vi "Re-Range.vi"(8 "error in (no error)":errorcluster, 10 "Config in":T1, 11 "DMM Driver in":refnum<class "DMM Driver.lvclass">) -> (0 "error out":errorcluster, 1 "Success?":bool, 2 "Config out":T1, 3 "DMM Driver out":refnum<class "DMM Driver.lvclass">)   [LabVIEW 2020, in "DMM.lvlib" / "DMM Driver.lvclass"]
doc: "Re-range the DMM using autorange and single measure. The autoranged measurement is discarded."
uses:
  DMM Driver.lvclass
  Controls/Ctl_DigitResolution.ctl
  DMM.lvlib
  Controls/Ctl_Function.ctl
  Controls/Community/Ctl_Config.ctl
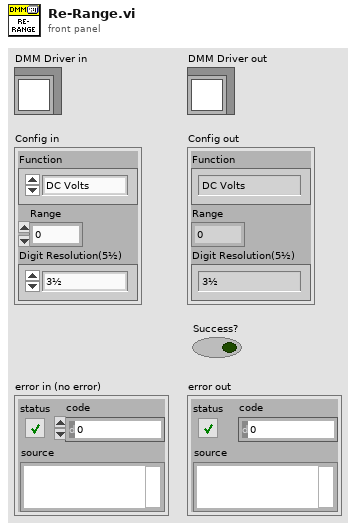
[diagram p1: front panel]
types:
  T1 = typedef "DMM.lvlib/Ctl_Config.ctl" = cluster{"Function":T2, "Range":dbl, "Digit Resolution(5½)":T3}
  T2 = typedef "DMM.lvlib/Ctl_Function.ctl" = enum8{"DC Volts", "AC Volts", "DC Current", "AC Current", "2-wire Resistance", "4-wire Resistance", "Diode", "Frequency", "Period", "AC Volts DC Coupled", "Capacitance", "Inductance", "Temperature"}
  T3 = typedef "DMM.lvlib/Ctl_DigitResolution.ctl" = enum8{"3½", "4½", "5½", "6½", "7½"}
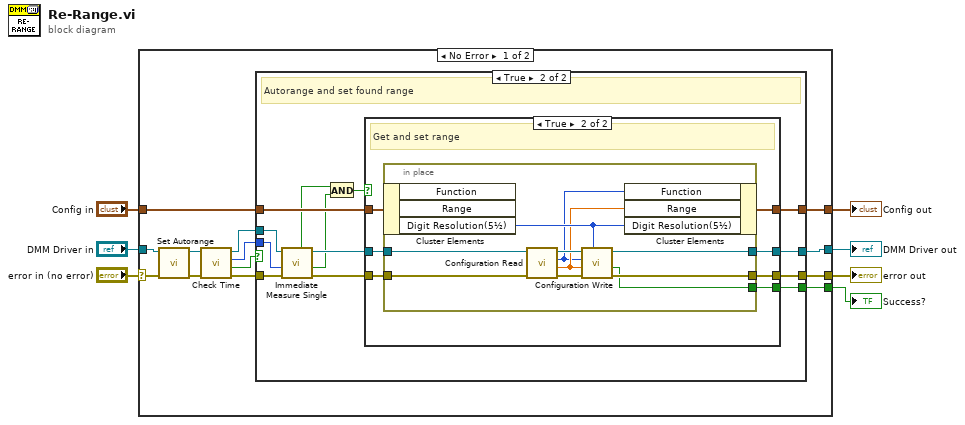
[diagram p0: block diagram]
diagram:
  n1 = case shown="No Error" "error in (no error)" {
    selector: "error in (no error)" -> [w18 w58]
    tunnel: [w20 w59] -> w7
    tunnel: "Config in" -> [w19 w59]
    tunnel: "DMM Driver in" -> [w17 w57]
    tunnel: [w16 _] -> w3
    tunnel: [w15 w57] -> w2
    tunnel: [w14 w58] -> w1
    frame No Error {
      n2 = call-dynamic "Set Autorange.vi"("error in (no error)"=w18, "DMM Driver in"=w17) -> ("error out"=w11:errorcluster, "DMM Driver out"=w8:refnum<class "DMM Driver.lvclass">)  [unwired: 8 in]
      n3 = call "Check Time.vi"("error in (no error)"=w11, "DMM Driver in"=w8) -> ("error out"=w10:errorcluster, "Time OK?"=w12:bool, "Remaining Time"=w13:i32, "DMM Driver out"=w9:refnum<class "DMM Driver.lvclass">)  [unwired: 6 in]
      n4 = case shown="True" w12 {
        tunnel: w9 -> [w22 w36]
        tunnel: w10 -> [w23 w35]
        tunnel: w13 -> [_ w34]
        tunnel: [w23 w31] -> w14
        tunnel: [w22 w30] -> w15
        tunnel: [_ w29] -> w16
        tunnel: w19 -> [w21 w28]
        tunnel: [w21 w27] -> w20
        frame False {
          # "Out of Time"
        }
        frame True {
          # "Autorange and set found range"
          n5 = call-dynamic "Immediate Measure Single.vi"("error in (no error)"=w35, "Max Time (-1ms)"=w34, "DMM Driver in"=w36) -> ("error out"=w32:errorcluster, "Valid measurement?"=w25:bool, "DMM Driver out"=w33:refnum<class "DMM Driver.lvclass">, "Finished?"=w26:bool)  [unwired: 4 in, 1 out]
          n6 = And(x=w26, y=w25) -> (x .and. y?=w24:bool)
          n7 = case shown="True" w24 {
            tunnel: w33 -> [w39 w46]
            tunnel: w32 -> [w37 w45]
            tunnel: [w37 w44] -> w31
            tunnel: [w39 w43] -> w30
            tunnel: [_ w42] -> w29
            tunnel: w28 -> [w38 w41]
            tunnel: [w38 w40] -> w27
            frame False {
              # "Autorange measure failed - Abort measure"
            }
            frame True {
              # "Get and set range"
              n8 = in-place {
                in-place-border: w46 -> [w56]
                in-place-border: w45 -> [w55]
                in-place-border: [w52] -> w44
                in-place-border: [w51] -> w43
                in-place-border: [w50] -> w42
                n9 = in-place-cluster #1(w41) -> ("Digit Resolution(5½)"=w49:T3)  [unwired: 2 out]
                n10 = call-dynamic "Configuration Read.vi"("error in (no error)"=w55, "DMM Driver in"=w56) -> ("error out"=w53:errorcluster, "Range"=w48:dbl, "Function"=w47:T2, "DMM Driver out"=w54:refnum<class "DMM Driver.lvclass">)  [unwired: 5 in, 1 out]
                n11 = call "Configuration Write.vi"("Digit Resolution(5½)"=w49, "error in (no error)"=w53, "Range"=w48, "Function"=w47, "DMM Driver in"=w54) -> ("error out"=w52:errorcluster, "Success?"=w50:bool, "DMM Driver out"=w51:refnum<class "DMM Driver.lvclass">)  [unwired: 4 in]
                n12 = in-place-cluster #1("Function"=w47, "Range"=w48, "Digit Resolution(5½)"=w49) -> (w40:T1)
              }
            }
          }
        }
      }
    }
    frame Error {
    }
  }
  "Config out" <- w7
  "Success?" <- w3
  "DMM Driver out" <- w2
  "error out" <- w1
